vi "Teleop_Calc_Toggle.vi"(0 "Init Value":dbl=0.8, 7 "Toggle Value":dbl, 11 "InButton":bool) -> (8 "Output":dbl)   [LabVIEW 2016]
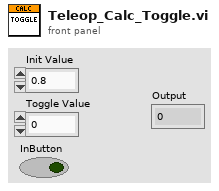
[diagram p1: front panel]
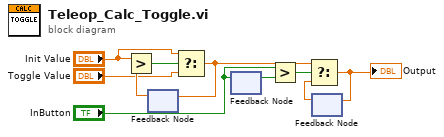
[diagram p0: block diagram]
diagram:
  n1 = feedback #1() -> (w8:dbl)  [unwired: 1 in]
  n2 = Greater?(x="Init Value", y=w8) -> (0:w7:bool)
  n3 = Select(t="Init Value", s=w7, f="Toggle Value") -> (s? t:f=w4:dbl)
  n4 = feedback-in #1(w4) -> ()
  n5 = feedback-in #2("InButton") -> ()
  n6 = feedback #2() -> (w10:bool)  [unwired: 1 in]
  n7 = Greater?(x="InButton", y=w10) -> (0:w6:bool)
  n8 = feedback #3() -> (w5:dbl)  [unwired: 1 in]
  n9 = Select(t=w4, s=w6, f=w5) -> (s? t:f=w3:dbl)
  "Output" <- w3
  n10 = feedback-in #3(w3) -> ()
